vi "EnqueueErrorMessage.vi"(8 "error in (no error)":errorcluster, 11 "message out":T1) -> (0 "error out":errorcluster)   [LabVIEW 2017, in "programControl.lvlib"]
uses:
  programControl.lvlib
  ErrorMonitor/Queue/TypeDefs/message.ctl
  Queue/TypeDefs/message.ctl
  ErrorMonitor/ErrorMonitor.lvlib
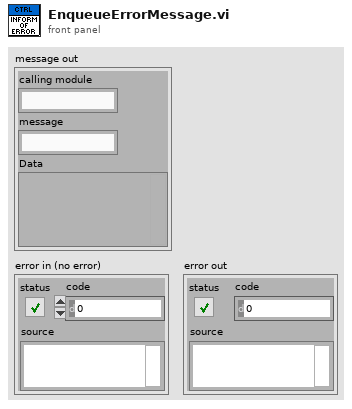
[diagram p1: front panel]
types:
  T1 = typedef "ErrorMonitor.lvlib/message.ctl" = cluster{"calling module":string, "message":string, "Data":variant}
  T2 = typedef "programControl.lvlib/message.ctl" = cluster{"calling module":string, "message":string, "Data":variant}
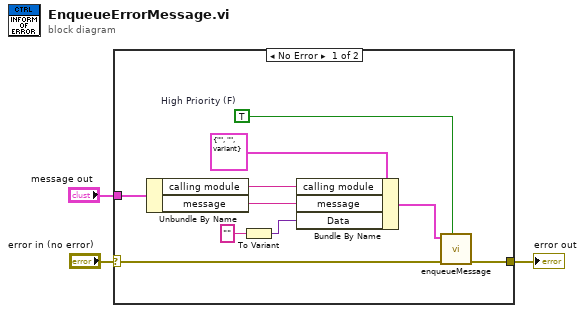
[diagram p0: block diagram]
diagram:
  n1 = case shown="No Error" "error in (no error)" {
    selector: "error in (no error)" -> [w12 w14]
    tunnel: [w13 w14] -> w3
    tunnel: "message out" -> [w11 _]
    frame No Error {
      w4 = TRUE  # High Priority (F)
      n2 = Unbundle By Name(w11) -> ("calling module"=w9:string, "message"=w8:string)
      n3 = To Variant(anything="") -> (Variant=w6:variant)
      n4 = Bundle By Name(cluster=T2 {"calling module"="", "message"="", "Data"=variant} ("message in"), "calling module"=w9, "message"=w8, "Data"=w6) -> (w5:T2)
      n5 = call "enqueueMessage.vi"("High Priority (F)"=w4, "error in (no error)"=w12, "element"=w5) -> ("error out"=w13:errorcluster)  [unwired: 8 in]
    }
    frame Error {
    }
  }
  "error out" <- w3
